vi "One Point Crossover.vi"(10 "Parent 1 in":T1, 11 "Parent 2 in":T1) -> (2 "Child 1 out":T1, 3 "Child 2 Out":T1)   [LabVIEW 2013, in "GA.lvclass"]
uses:
  GA.lvclass
  Controls/Solution_GA.ctl
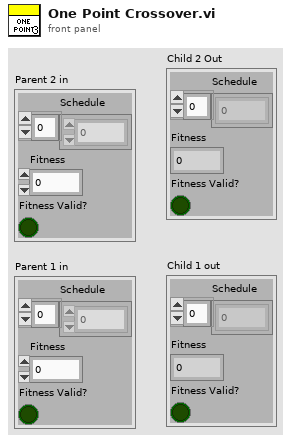
[diagram p1: front panel]
types:
  T1 = typedef "Solution_GA.ctl" = cluster{"Schedule":u16[], "Fitness":u16, "Fitness Valid?":bool}
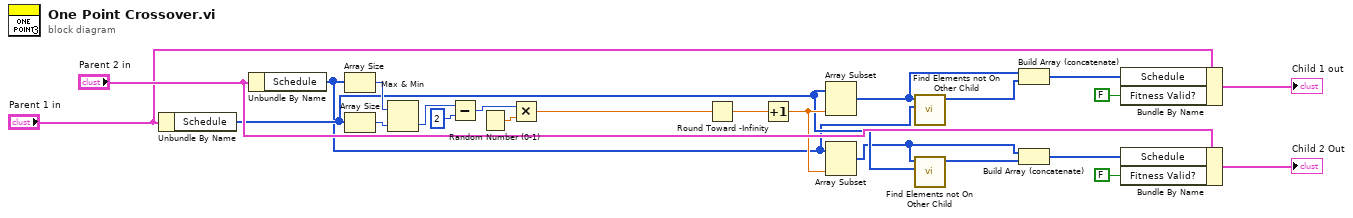
[diagram p0: block diagram]
diagram:
  n1 = Unbundle By Name("Parent 1 in") -> ("Schedule"=w10:u16[])
  n2 = Unbundle By Name("Parent 2 in") -> ("Schedule"=w9:u16[])
  n3 = Array Size(array=w9) -> (size(s)=w19:i32)
  n4 = Array Size(array=w10) -> (size(s)=w18:i32)
  n5 = Max & Min(x=w19, y=w18) -> (min(x,y)=w15:i32)  [unwired: 1 out]
  n6 = Subtract(x=w15, y=2) -> (x-y=w13:i32)
  n7 = Random Number (0-1)() -> (number: 0 to 1=w17:dbl)
  n8 = Multiply(x=w13, y=w17) -> (x*y=w16:dbl)
  n9 = Round Toward -Infinity(1:w16) -> (0:w12:dbl)
  n10 = Increment(x=w12) -> (x+1=w11:dbl)
  n11 = Array Subset(array=w10, length=w11) -> (w6:u16[])  [unwired: 1 in]
  n12 = Array Subset(array=w9, length=w11) -> (w8:u16[])  [unwired: 1 in]
  n13 = call "Find Elements not On Other Child.vi"("Schedule"=w9, "Sub Array"=w6) -> ("Elements to append"=w5:i32[])  [unwired: 9 in]
  n14 = call "Find Elements not On Other Child.vi"("Schedule"=w10, "Sub Array"=w8) -> ("Elements to append"=w7:i32[])  [unwired: 9 in]
  n15 = Build Array (concatenate)(w6, w5) -> (w2:i32[])
  n16 = Build Array (concatenate)(w8, w7) -> (w4:i32[])
  n17 = Bundle By Name(cluster="Parent 1 in", "Schedule"=w2, "Fitness Valid?"=FALSE) -> (→"Child 1 out":T1)
  n18 = Bundle By Name(cluster="Parent 2 in", "Schedule"=w4, "Fitness Valid?"=FALSE) -> (→"Child 2 Out":T1)
